vi "DataTreeCtrl setRefnum.vi"(7 "listDataInfo":refnum<vi>, 8 "error in (no error)":errorcluster, 9 "File Tree":refnum<vi>, 10 "Document Tree":refnum<vi>, 11 "DataTreeCtrl in":refnum<class "DataTreeCtrl.lvclass">) -> (0 "error out":errorcluster, 3 "DataTreeCtrl out":refnum<class "DataTreeCtrl.lvclass">)   [LabVIEW 2018, in "DataTreeCtrl.lvclass"]
uses:
  DataTreeCtrl.lvclass
  DataTreeCtrl.lvclass/DataTreeCtrl.ctl
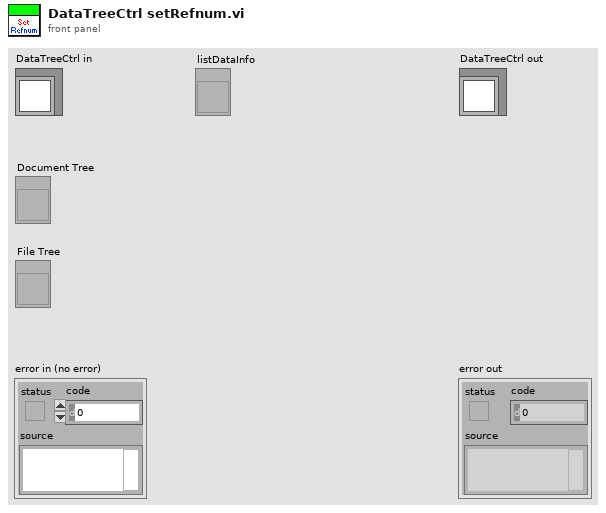
[diagram p1: front panel]
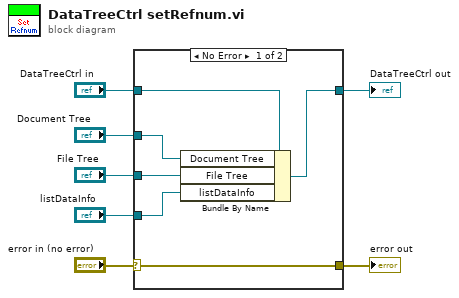
[diagram p0: block diagram]
diagram:
  n1 = case shown="No Error" "error in (no error)" {
    selector: "error in (no error)" -> [w13 w15]
    tunnel: [w13 w15] -> w6
    tunnel: [w9 w14] -> w4
    tunnel: "DataTreeCtrl in" -> [w12 w14]
    tunnel: "Document Tree" -> [w11 _]
    tunnel: "File Tree" -> [w10 _]
    tunnel: "listDataInfo" -> [w8 _]
    frame No Error {
      n2 = Bundle By Name(cluster=w12, "Document Tree"=w11, "File Tree"=w10, "listDataInfo"=w8) -> (w9:refnum<class "DataTreeCtrl.lvclass">)
    }
    frame Error {
    }
  }
  "error out" <- w6
  "DataTreeCtrl out" <- w4
